vi "collectdata.vi"(8 "error IO":errorcluster, 9 "Number of modules":T1, 10 "millisecond timer value":u32, 11 "DAQmx Task Name":refnum<k21>) -> (0 "error out":errorcluster, 2 "mod2":u16[](array[numeric]), 3 "listmodedata":u16[](array[numeric]), 4 "labview time":dbl, 5 "pulses recieved":u32, 6 "zero values?":bool, 7 "Total time [s]":dbl)   [LabVIEW 2016]
doc: "Gets the total nubmer of pulser events sent to the pxi chassis as well as \ndownloads pixie listmode data"
uses:
  realtime data/pixie vis/controls/number of modules.ctl
  <vilib>/DAQmx/read.llb/DAQmx Read (Counter U32 1Chan 1Samp).vi
  <vilib>/DAQmx/miscellaneous.llb/DAQmx Fill In Error Info.vi
panel:
  out "pixie runtime":dbl
  out "pixie internal lt":dbl
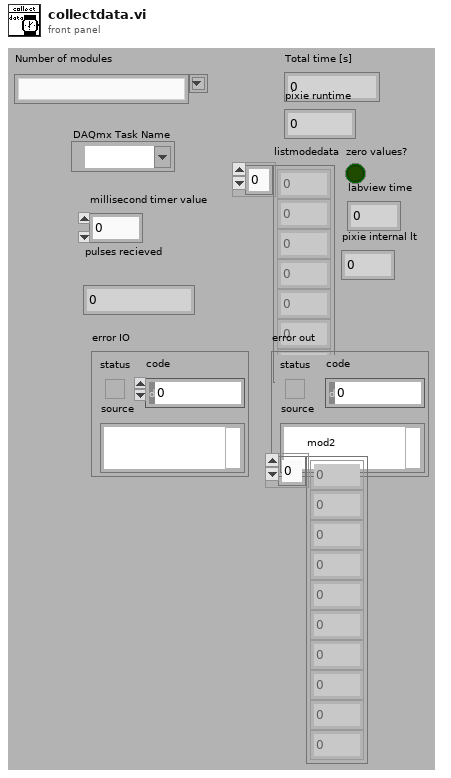
[diagram p1: front panel]
types:
  T1 = typedef "number of modules.ctl" = string
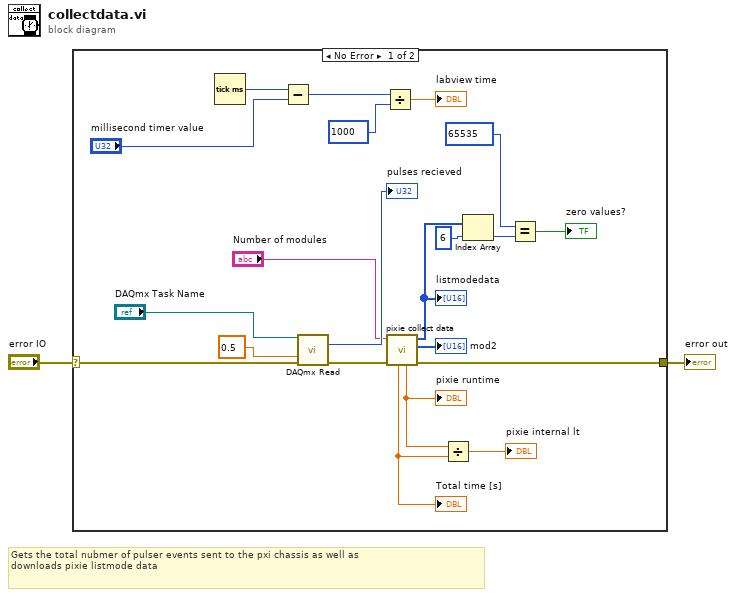
[diagram p0: block diagram]
diagram:
  # "Gets the total nubmer of pulser events sent to the pxi chassis as well as \ndownloads pixie listmode data"
  n1 = case shown="No Error" "error IO" {
    selector: "error IO" -> [w16 w24]
    tunnel: [w21 w24] -> w2
    frame No Error {
      n2 = Tick Count (ms)() -> (millisecond timer value=w19:u32)
      n3 = Subtract(x=w19, y="millisecond timer value") -> (x-y=w15:u32)
      n4 = call-poly <vilib>:"DAQmx Read.vi"("task/channels in"="DAQmx Task Name", "timeout"=0.5, "error in"=w16) -> ("data"=→"pulses recieved":u32, "error out"=w22:errorcluster)  [unwired: 10 in, 1 out]
      n5 = Divide(x=w15, y=u32 1000) -> (x/y=→"labview time":dbl)
      n6 = call "pixie collect data.vi"("error in"=w22, "Number of modules"="Number of modules") -> ("error out"=w21:errorcluster, "mod2"=→"mod2":u16[], "mode 0"=w5:u16[], "pixie runtime"=w12:dbl, "Total time [s]"=w11:dbl)  [unwired: 5 in]
      "listmodedata" <- w5
      "Total time [s]" <- w11
      "pixie runtime" <- w12
      n7 = Divide(x=w12, y=w11) -> (x/y=→"pixie internal lt":dbl)
      n8 = Index Array(array=w5, index=6) -> (element=w7:u16)
      n9 = Equal?(x=u16 65535, y=w7) -> (x = y?=→"zero values?":bool)
    }
    frame Error {
    }
  }
  "error out" <- w2
